vi "color.vi"(0 "Match Saturation Threshold (Color Matching 1)":i32=80, 7 "error in":errorcluster) -> (20 "Match Flag (Color Matching 1)":bool[](array[boolean]), 21 "Match Score (Color Matching 1)":i32[](array[numeric]), 27 "error out":errorcluster)   [LabVIEW 2015]
uses:
  <vilib>/vision/driver/NI_Vision_Acquisition_Software.lvlib
  <vilib>/vision/NI_Vision_Development_Module.lvlib
panel:
  out "Image Out":T1(plugin-control)
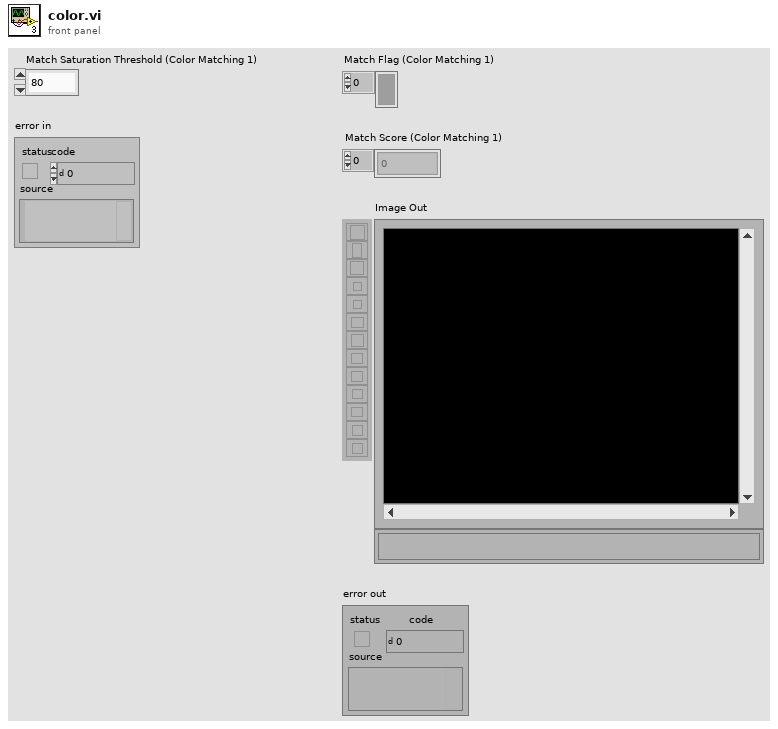
[diagram p1: front panel]
types:
  T1 = typedef "IMAQ Image.ctl" = refnum<image>
  T2 = cluster{"Global Rectangle":i32[], "Contours":cluster{"ID":enum32{"External", "Internal"}, "Type":u32, "Coordinates":i32[]}[]}
  T3 = typedef "IMAQdx.ctl" = refnum<k21>
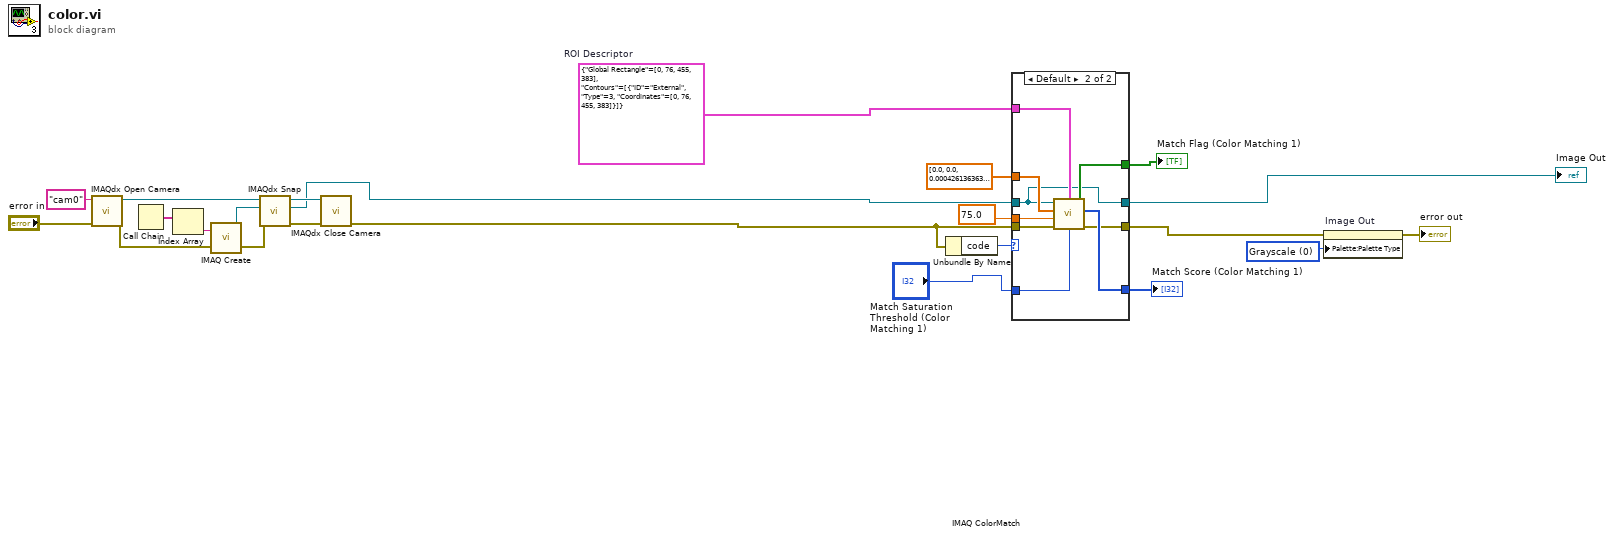
[diagram p0: block diagram]
diagram:
  w1 = u32 0 items=["Grayscale", "Binary", "Gradient", "Rainbow", "Temperature", "User Defined", "Binary 16 Bit", "Gradient 16 Bit", "Rainbow 16 Bit", "Temperature 16 Bit", "User Defined 16 Bit"] ("Palette Type")
  w5 = T2 {"Global Rectangle"=[0, 76, 455, 383], "Contours"=[{"ID"=enum."External", "Type"=3, "Coordinates"=[0, 76, 455, 383]}]}  # ROI Descriptor
  n1 = call <vilib>:"IMAQdx Open Camera.vi"("error in"="error in", "Session In"="cam0" ("Interface Name")) -> ("error out"=w22:errorcluster, "Session Out"=w16:T3)  [unwired: 1 in, 7 out]
  n2 = Call Chain() -> (call chain=w14:string[])
  n3 = Index Array(array=w14) -> (element=w13:string)  [unwired: 1 in]
  n4 = call "IMAQ Create"("Image Name"=w13, "error in (no error)"=w22) -> ("New Image"=w18:T1, "error out"=w17:errorcluster)  [unwired: 2 in, 1 out]
  n5 = call <vilib>:"IMAQdx Snap.vi"("error in"=w17, "Image In"=w18, "Session In"=w16) -> ("error out"=w20:errorcluster, "Image Out"=w7:T1, "Session Out"=w21:T3)  [unwired: 6 out]
  n6 = call <vilib>:"IMAQdx Close Camera.vi"("error in"=w20, "Session In"=w21) -> ("error out"=w19:errorcluster)  [unwired: 9 out]
  n7 = Unbundle By Name(w19) -> ("code"=w4:i32)
  n8 = case shown="Default" w4 {
    tunnel: 75.0 ("Minimum Match Score") -> [_ w33]
    tunnel: "Match Saturation Threshold (Color Matching 1)" -> [_ w32]
    tunnel: dbl[] [0.0, 0.0, 0.0004261363636363636, 0.0, 0.007244318181818182, 0.020170454545454547, 0.06491477272727272, 0.9058238636363637, 0.00014204545454545454, 0.0, 0.0, 0.0, 0.0, 0.0, 0.0, 0.001278409090909091] ("Color Spectrum") -> [_ w31]
    tunnel: [_ w30] -> w9
    tunnel: [_ w29] -> w8
    tunnel: w7 -> [w24 w25]
    tunnel: w19 -> [_ w28]
    tunnel: [_ w27] -> w6
    tunnel: w5 -> [_ w26]
    tunnel: [w24 w25] -> w2
    frame -1074396199, -1074396198 {
      # "Discard\nCoordinate\nSystem Error"
    }
    frame Default {
      n9 = call "IMAQ ColorMatch"("ROI Descriptor"=w26, "Image"=w25, "Color Spectrum"=w31, "Match Saturation Threshold"=w32, "Minimum Match Score"=w33, "error in (no error)"=w28) -> ("Match Flag"=w30:bool[], "Match Score"=w29:i32[], "error out"=w27:errorcluster)  [unwired: 1 out]
    }
  }
  "Match Flag (Color Matching 1)" <- w9
  "Match Score (Color Matching 1)" <- w8
  "Image Out" <- w2
  n10 = property on="Image Out" class="ImageControl"(error in=w6, "Palette:Palette Type"=w1) -> (error out=→"error out":errorcluster)  [unwired: 1 in, 1 out]
